vi "scale.vi"(11 "Int result array":i16[](array[numeric])) -> (3 "Scaled result":dbl[](array[numeric]))   [LabVIEW 2015]
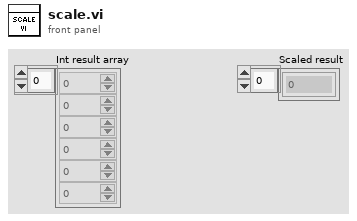
[diagram p1: front panel]
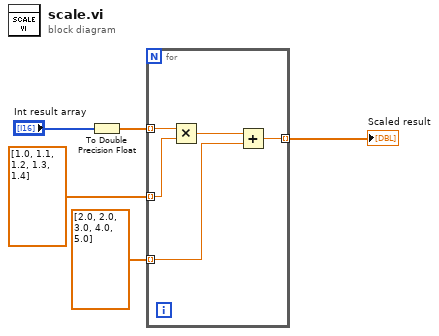
[diagram p0: block diagram]
diagram:
  n1 = To Double Precision Float(number="Int result array") -> (double precision float=w4:dbl[])
  n2 = for {
    tunnel: w4 -> [w10] mode=indexing
    tunnel: dbl[] [1.0, 1.1, 1.2, 1.3, 1.4] -> [w9] mode=indexing
    tunnel: dbl[] [2.0, 2.0, 3.0, 4.0, 5.0] -> [w7] mode=indexing
    tunnel: [w6] -> w1 mode=indexing
    n3 = Multiply(x=w10, y=w9) -> (x*y=w8:dbl)
    n4 = Add(x=w8, y=w7) -> (x+y=w6:dbl)
  }
  "Scaled result" <- w1
